vi "VI_get app kind.vi"(8 "error in (no error)":errorcluster, 11 "VI in":refnum<vi>) -> (0 "error out":errorcluster, 2 "App.Kind":T1(ring), 3 "VI out":refnum<vi>)   [LabVIEW 2015]
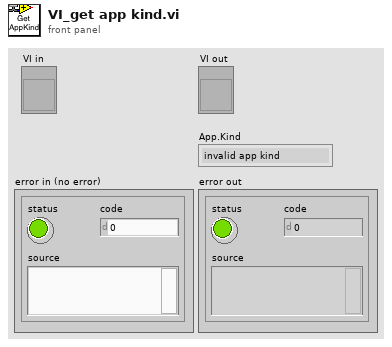
[diagram p1: front panel]
types:
  T1 = enum32{"invalid app kind", "Development System", "Run Time System", "Student Edition", "Embedded LabVIEW", "Evaluation", "Custom"}
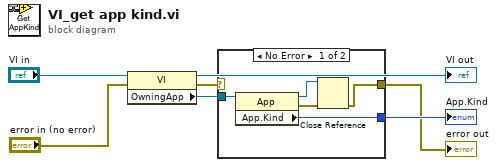
[diagram p0: block diagram]
diagram:
  n1 = property class="VI"(reference="VI in", error in="error in (no error)") -> (reference out=→"VI out":refnum<vi>, error out=w6:errorcluster, "OwningApp"=w4:refnum<vi>)
  n2 = case shown="No Error" w6 {
    selector: w6 -> [_ w13]
    tunnel: w4 -> [w12 _]
    tunnel: [w9 _] -> w7
    tunnel: [w8 w13] -> w1
    frame No Error {
      n3 = property class="App"(reference=w12) -> (reference out=w11:refnum<vi>, error out=w10:errorcluster, "App.Kind"=w9:T1)  [unwired: 1 in]
      n4 = Close Reference(reference=w11, error in (no error)=w10) -> (error out=w8:errorcluster)
    }
    frame Error {
    }
  }
  "App.Kind" <- w7
  "error out" <- w1
